vi "Waveform Test V1.vi"() -> ()   [LabVIEW 2014]
uses:
  <vilib>/FPGAPlugInAG/PCIe-7841R/niLvFpga_Open_PCIe-7841R.vi
  <vilib>/Utility/error.llb/Error Cluster From Error Code.vi
  <vilib>/rvi/errors/niLvFpgaAdjustHostInterfaceError.vi
  <vilib>/FPGAPlugInAG/PCIe-7841R/niLvFpga_Run_PCIe-7841R.vi
  <vilib>/FPGAPlugInAG/PCIe-7841R/niLvFpga_Abort_PCIe-7841R.vi
  <vilib>/FPGAPlugInAG/PCIe-7841R/niLvFpga_Close_PCIe-7841R.vi
  <vilib>/rvi/interface/nirviOpenFPGA/nirviOpenFPGA.xnode
  FPGA Bitfiles/MainSTEDFPGAProj_FPGATarget_WaveformandLaser_Z6o9JHl3Kiw.lvbitx
  <vilib>/rvi/interface/nirviReadWriteControl/nirviReadWriteControl.xnode
  <vilib>/rvi/interface/nirviMethod/nirviMethod.xnode
  <vilib>/rvi/interface/nirviCloseFPGA/nirviCloseFPGA.xnode
  NiFpgaLv.dll
panel:
  in  "STOP WF":bool
  in  "Run WF":bool
  in  "stop":bool
  in  "Offset (V)":dbl
  in  "Amplitude (V)":dbl
  out "XY Graph":cluster{dbl[], dbl[]}[](graph)
  in  "Number of Samples":i32
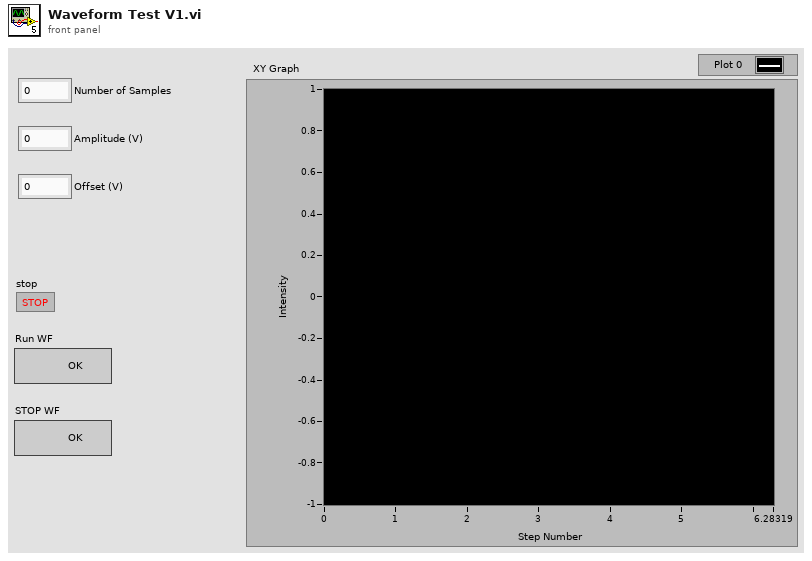
[diagram p1: front panel]
types:
  T1 = cluster{"Res Mirror Amp (I16)":i16, "Res Mirror Mute":bool}
  T2 = cluster{"AOM (Pin 51 AO4)":i16, "Beam Blanking":bool}
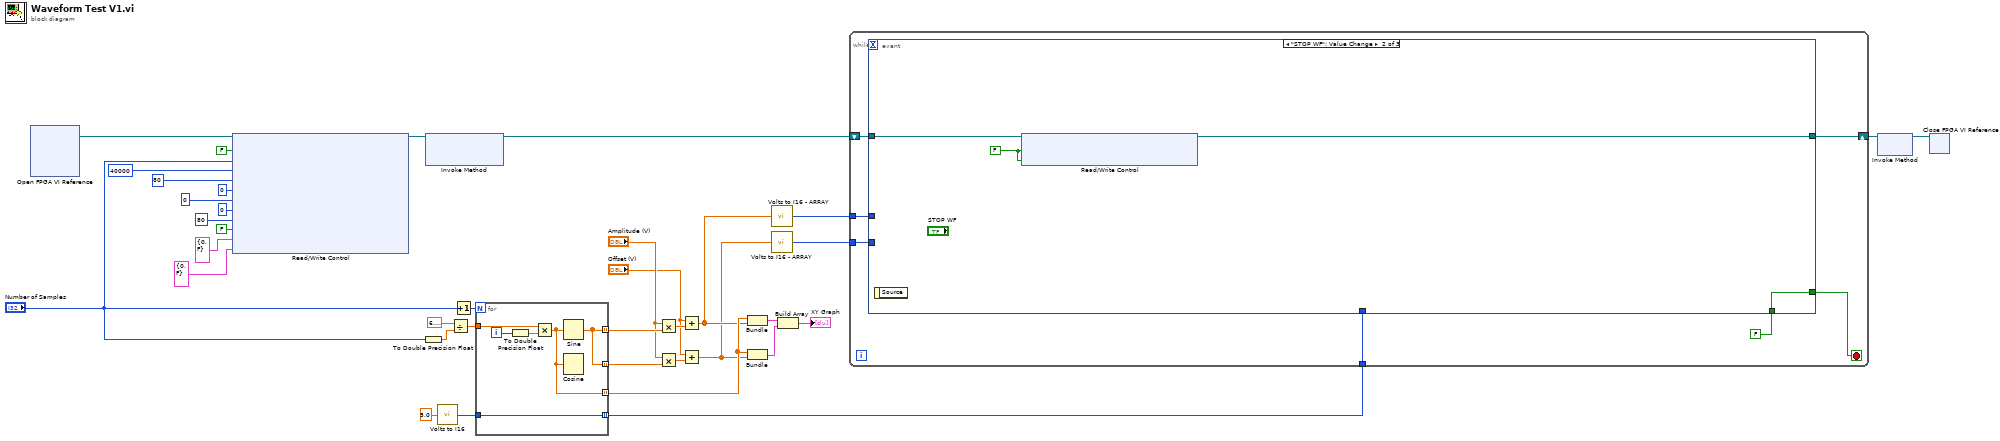
[diagram p0: block diagram]
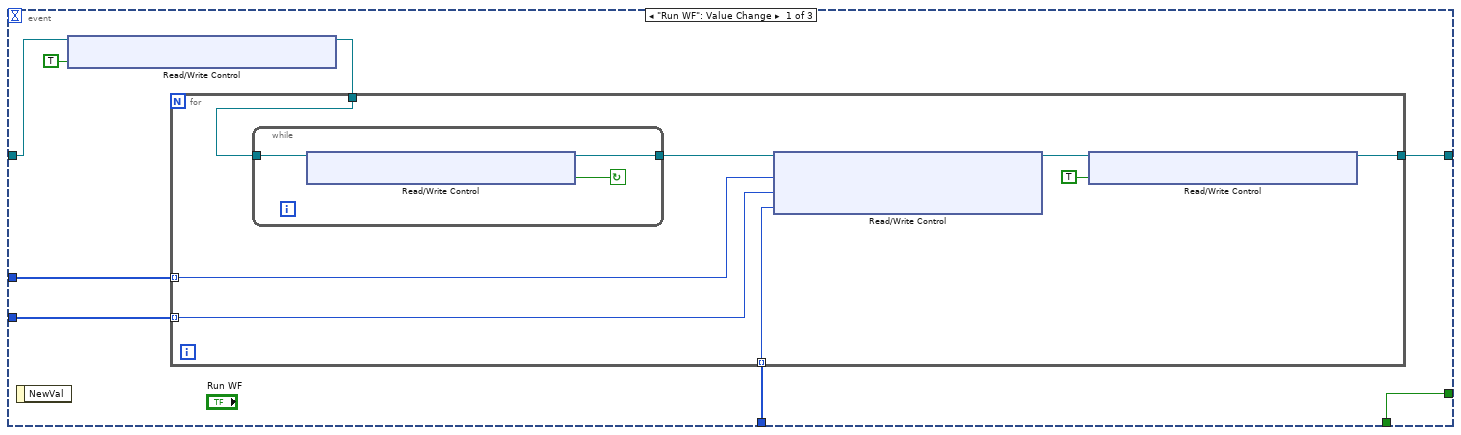
[diagram p2: hidden frame]
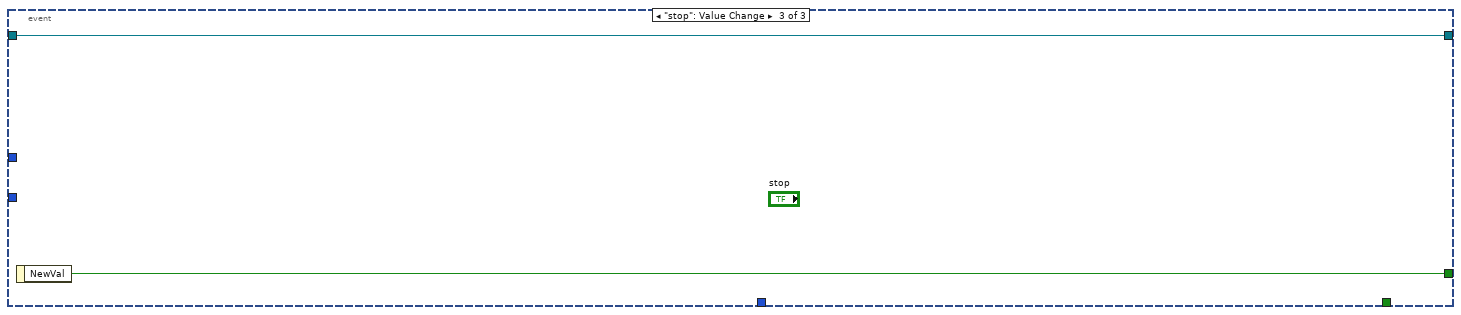
[diagram p3: hidden frame]
diagram:
  n1 = xnode "Open FPGA VI Reference"() -> ("FPGA VI Reference Out"=w23:refnum<k20>)  [unwired: 2 in, 1 out]
  n2 = xnode "Read/Write Control"("FPGA VI Reference In"=w23, "Host Data Loaded"=FALSE, "Waveform Length (Elements)"="Number of Samples", "Slow Axis 1 Delay (25 ns) Steps"=40000, "Fast Axis Sample Period (Ticks)"=u32 80, "Slow Axis 2 Delay (25 ns) Steps"=0, "Scanning Mode"=u8 0, "Unused Axis Offset"=i16 0, "Slow Axis 1 Sample Period (Ticks)"=u32 80, "Start Waveforms"=FALSE, "775 AOM"=T2 {"AOM (Pin 51 AO4)"=0, "Beam Blanking"=FALSE}, "Resoance Mirror"=T1 {"Res Mirror Amp (I16)"=0, "Res Mirror Mute"=FALSE}) -> ("FPGA VI Reference Out"=w22:refnum<k20>)  [unwired: 1 in, 1 out]
  n3 = To Double Precision Float(number="Number of Samples") -> (double precision float=w36:dbl)
  n4 = xnode "Invoke Method"("FPGA VI Reference In"=w22) -> ("FPGA VI Reference Out"=w21:refnum<k20>)  [unwired: 2 in, 1 out]
  n5 = call "Volts to I16.vi"("Voltage (V)"=5.0) -> ("I16"=w14:i16)  [unwired: 14 in]
  n6 = Divide(x=6.283185307179586, y=w36) -> (x/y=w35:dbl)
  n7 = Increment(x="Number of Samples") -> (x+1=w30:i32)
  n8 = for {
    N: w30 -> [_]
    tunnel: w35 -> [w43]
    tunnel: [w38] -> w29 mode=indexing
    tunnel: [w38] -> w26 mode=indexing
    tunnel: [w40] -> w34 mode=indexing
    tunnel: w14 -> [w39]
    tunnel: [w39] -> w13 mode=indexing
    i -> [w42]
    n9 = To Double Precision Float(number=w42) -> (double precision float=w41:dbl)
    n10 = Multiply(x=w43, y=w41) -> (x*y=w40:dbl)
    n11 = Sine(x=w40) -> (sin(x)=w38:dbl)
    n12 = Cosine(x=w40) -> ()  [unwired: 1 out]
  }
  n13 = Multiply(x="Amplitude (V)", y=w29) -> (x*y=w28:dbl[])
  n14 = Multiply(x="Amplitude (V)", y=w26) -> (x*y=w27:dbl[])
  n15 = Add(x="Offset (V)", y=w28) -> (x+y=w19:dbl[])
  n16 = Add(x="Offset (V)", y=w27) -> (x+y=w17:dbl[])
  n17 = Bundle(w34, w19) -> (w33:cluster{dbl[], dbl[]})  [unwired: 1 in]
  n18 = Bundle(w34, w17) -> (w32:cluster{dbl[], dbl[]})  [unwired: 1 in]
  n19 = call "Volts to I16 - ARRAY.vi"("Voltage (V)"=w19) -> ("I16"=w18:i16[])  [unwired: 14 in]
  n20 = call "Volts to I16 - ARRAY.vi"("Voltage (V)"=w17) -> ("I16"=w15:i16[])  [unwired: 14 in]
  n21 = Build Array(w33, w32) -> (→"XY Graph":cluster{dbl[], dbl[]}[])
  n22 = while {
    tunnel: w18 -> [w49]
    tunnel: w15 -> [w48]
    tunnel: w13 -> [w47]
    shift-right: [w46] -> w1
    shift-left: w21 -> [w50]
    stop <- w45 stop-if-true
    n23 = event shown="[1] \"STOP WF\": Value Change" {
      selector: _ -> [_ _ _]
      dyn-events: _ -> [_ _ _]
      timeout: _ -> [_ _ _]
      tunnel: w50 -> [w54 w73 w74]
      tunnel: w49 -> [w58 _ _]
      tunnel: w48 -> [w57 _ _]
      tunnel: w47 -> [w56 _ _]
      tunnel: [w55 w72 w74] -> w46
      tunnel: [w51 w70 w75] -> w45
      tunnel: FALSE -> [w51 w70 _]
      event "Run WF": Value Change {
        n24 = event-data() -> ()  [unwired: 1 in, 1 out]
        n25 = xnode "Read/Write Control"("FPGA VI Reference In"=w54, "Start Waveforms"=TRUE) -> ("FPGA VI Reference Out"=w53:refnum<k20>)  [unwired: 1 in, 1 out]
        n26 = for {
          tunnel: w58 -> [w66] mode=indexing
          tunnel: w57 -> [w61] mode=indexing
          tunnel: [w62] -> w55
          tunnel: w56 -> [w60] mode=indexing
          tunnel: w53 -> [w59]
          n27 = while {
            tunnel: w59 -> [w69]
            tunnel: [w68] -> w63
            stop <- w67 continue-if-true
            n28 = xnode "Read/Write Control"("FPGA VI Reference In"=w69) -> ("FPGA VI Reference Out"=w68:refnum<k20>, "Host Data Loaded"=w67:bool)  [unwired: 1 in, 1 out]
          }
          n29 = xnode "Read/Write Control"("FPGA VI Reference In"=w63, "Fast Axis Waveform Element"=w66, "Slow Axis Waveform 1 Element"=w61, "Slow Axis Waveform 2 Element"=w60) -> ("FPGA VI Reference Out"=w65:refnum<k20>)  [unwired: 1 in, 1 out]
          n30 = xnode "Read/Write Control"("FPGA VI Reference In"=w65, "Host Data Loaded"=TRUE) -> ("FPGA VI Reference Out"=w62:refnum<k20>)  [unwired: 1 in, 1 out]
        }
      }
      event "STOP WF": Value Change {
        w71 = FALSE ("Start Waveforms")
        n31 = event-data() -> ()  [unwired: 1 in, 1 out]
        n32 = xnode "Read/Write Control"("FPGA VI Reference In"=w73, "Start Waveforms"=w71, "Host Data Loaded"=w71) -> ("FPGA VI Reference Out"=w72:refnum<k20>)  [unwired: 1 in, 1 out]
      }
      event "stop": Value Change {
        n33 = event-data() -> ("NewVal"=w75:bool)  [unwired: 1 in]
      }
    }
  }
  n34 = xnode "Invoke Method"("FPGA VI Reference In"=w1) -> ("FPGA VI Reference Out"=w20:refnum<k20>)  [unwired: 1 in, 1 out]
  n35 = xnode "Close FPGA VI Reference"("FPGA VI Reference In"=w20) -> ()  [unwired: 1 in, 1 out]
